vi "PXI-Prime AO.vi"(0 "AO Tasks":T1[](array[typedef]), 1 "error in":errorcluster) -> (2 "AO Tasks out":T1[](array[typedef]), 3 "AO Waveforms":dbl[][](array[numeric]), 4 "error out":errorcluster)   [LabVIEW 2020]
uses:
  Type Defs/Task Struct.ctl
  PXI Globals.vi
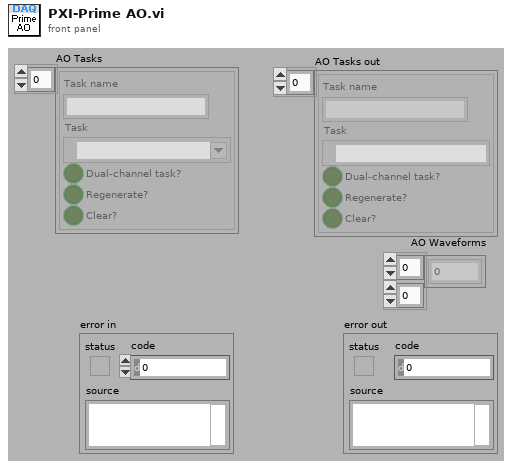
[diagram p1: front panel]
types:
  T1 = typedef "Task Struct.ctl" = cluster{"Task name":string, "Task":refnum<k21>, "Dual-channel task?":bool, "Regenerate?":bool, "Clear?":bool}
  T2 = typedef "Ramping Params.ctl" = cluster{"Ramp up?":bool, "Ramp down?":bool, "Ramp duration (msecs)":dbl, "Ramp type":enum16{"Linear", "Cos2"}}
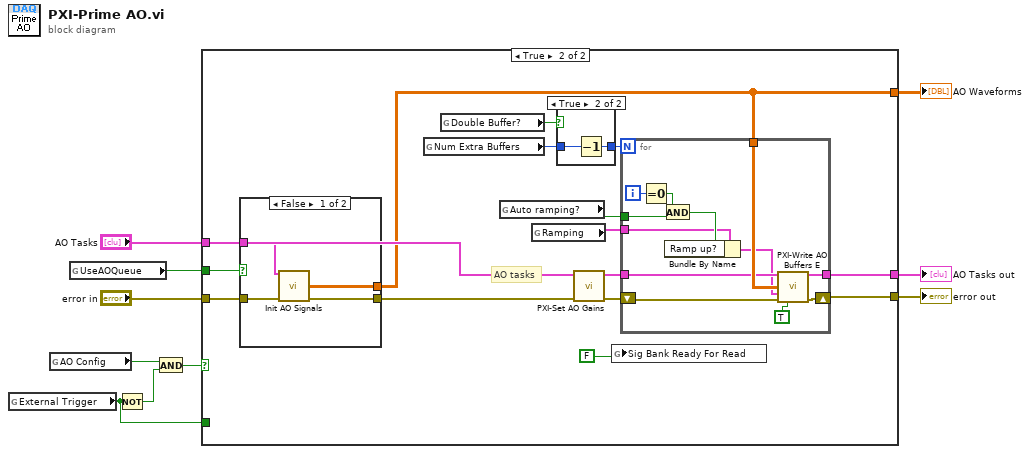
[diagram p0: block diagram]
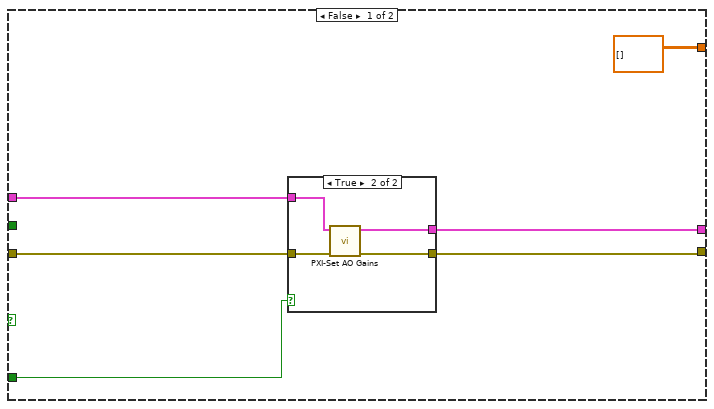
[diagram p2: hidden frame]
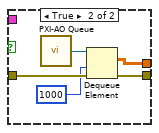
[diagram p4: hidden frame]
diagram:
  n1 = global read "PXI Globals.vi" "External Trigger"() -> (w4:bool)
  n2 = global read "PXI Globals.vi" "AO Config"() -> (w2:bool)
  n3 = global read "PXI Globals.vi" "UseAOQueue"() -> (w3:bool)
  n4 = Not(x=w4) -> (.not. x?=w5:bool)
  n5 = And(x=w2, y=w5) -> (x .and. y?=w1:bool)
  n6 = case shown="True" w1 {
    tunnel: "error in" -> [w14 w37]
    tunnel: [w13 w36] -> w8
    tunnel: "AO Tasks" -> [w15 w26]
    tunnel: [w12 w25] -> w9
    tunnel: [dbl[][] [] ("AO Waveforms") w24] -> w6
    tunnel: w4 -> [w11 _]
    tunnel: w3 -> [_ w23]
    frame False {
      n7 = case shown="True" w11 {
        tunnel: w15 -> [w18 w22]
        tunnel: w14 -> [w17 w21]
        tunnel: [w17 w20] -> w13
        tunnel: [w18 w19] -> w12
        frame False {
        }
        frame True {
          n8 = call "PXI-Set AO Gains.vi"("error in (no error)"=w21, "AO Tasks"=w22) -> ("error out"=w20:errorcluster, "AO Tasks out"=w19:T1[])  [unwired: 8 in]
        }
      }
    }
    frame True {
      # "AO tasks"
      n9 = case shown="False" w23 {
        tunnel: w37 -> [w41 w44]
        tunnel: [w40 w45] -> w33
        tunnel: w26 -> [w39 _]
        tunnel: [w38 w43] -> w24
        frame False {
          n10 = call "Init AO Signals.vi"("AO Tasks"=w39, "error in (no error)"=w41) -> ("AO Waveforms"=w38:dbl[][], "error out"=w40:errorcluster)  [unwired: 12 in]
        }
        frame True {
          n11 = call "PXI-AO Queue.vi"() -> ("Queue"=w46:refnum<queue>)  [unwired: 15 in]
          n12 = Dequeue Element(queue=w46, timeout in ms (-1)=1000, error in (no error)=w44) -> (element=w43:dbl[][], error out=w45:errorcluster)  [unwired: 2 out]
        }
      }
      n13 = global read "PXI Globals.vi" "Num Extra Buffers"() -> (w29:i32)
      n14 = global read "PXI Globals.vi" "Double Buffer?"() -> (w32:bool)
      n15 = global read "PXI Globals.vi" "Auto ramping?"() -> (w31:bool)
      n16 = global read "PXI Globals.vi" "Ramping"() -> (w30:T2)
      n17 = case shown="True" w32 {
        tunnel: [w47 w49] -> w34
        tunnel: w29 -> [w47 w48]
        frame False {
        }
        frame True {
          n18 = Decrement(x=w48) -> (x-1=w49:i32)
        }
      }
      n19 = call "PXI-Set AO Gains.vi"("error in (no error)"=w33, "AO Tasks"=w26) -> ("error out"=w28:errorcluster, "AO Tasks out"=w27:T1[])  [unwired: 8 in]
      n20 = global write "PXI Globals.vi" "Sig Bank Ready For Read"(FALSE) -> ()
      n21 = for {
        N: w34 -> [_]
        tunnel: w30 -> [w56]
        shift-right: [w61] -> w36
        shift-left: w28 -> [w55]
        tunnel: w31 -> [w53]
        tunnel: w24 -> [w57]
        tunnel: w27 -> [w54]
        tunnel: [w52] -> w25
        i -> [w60]
        n22 = Equal To 0?(x=w60) -> (x = 0?=w59:bool)
        n23 = And(x=w59, y=w53) -> (x .and. y?=w58:bool)
        n24 = Bundle By Name(cluster=w56, "Ramp up?"=w58) -> (w50:T2)
        n25 = call "PXI-Write AO Buffers E.vi"("AO Tasks"=w54, "AO Waveforms"=w57, "Ramping"=w50, "error in (no error)"=w55, "Force write"=TRUE) -> ("AO Tasks out"=w52:T1[], "error out"=w61:errorcluster)  [unwired: 9 in]
      }
    }
  }
  "AO Tasks out" <- w9
  "error out" <- w8
  "AO Waveforms" <- w6
